vi "Generate Intensities.vi"(9 "eta*cosalpha":dbl=-0.0303, 10 "Lorentzian Width":dbl=0.05, 11 "Numeric":dbl) -> (3 "Intensity":dbl)   [LabVIEW 2020]
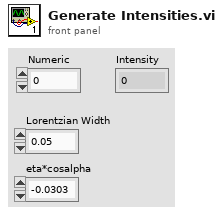
[diagram p1: front panel]
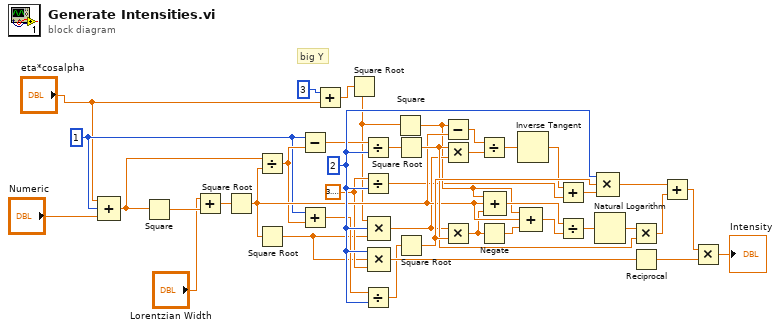
[diagram p0: block diagram]
diagram:
  w18 = 3.141592653589793
  w35 = 2
  w15 = 1
  # "big Y"
  n1 = Compound Arithmetic op=ADD("eta*cosalpha", w15, "Numeric") -> (w9:dbl)
  n2 = Square(x=w9) -> (x^2=w7:dbl)
  n3 = Add(x="Lorentzian Width", y=w7) -> (x+y=w8:dbl)
  n4 = Square Root(x=w8) -> (sqrt(x)=w29:dbl)
  n5 = Divide(x=w9, y=w29) -> (x/y=w16:dbl)
  n6 = Square Root(x=w29) -> (sqrt(x)=w3:dbl)
  n7 = Subtract(x=w15, y=w16) -> (x-y=w11:dbl)
  n8 = Add(x=w15, y=w16) -> (x+y=w10:dbl)
  n9 = Add(x=3, y="eta*cosalpha") -> (x+y=w19:dbl)
  n10 = Square Root(x=w19) -> (sqrt(x)=w5:dbl)
  n11 = Divide(x=w11, y=w35) -> (x/y=w14:dbl)
  n12 = Divide(x=w18, y=w35) -> (x/y=w24:dbl)
  n13 = Divide(x=w10, y=w35) -> (x/y=w13:dbl)
  n14 = Compound Arithmetic op=MULTIPLY(w5, w35, w3) -> (w27:dbl)
  n15 = Compound Arithmetic op=MULTIPLY(w35, w3, w18) -> (w17:dbl)
  n16 = Square(x=w5) -> (x^2=w26:dbl)
  n17 = Square Root(x=w14) -> (sqrt(x)=w34:dbl)
  n18 = Square Root(x=w13) -> (sqrt(x)=w36:dbl)
  n19 = Subtract(x=w26, y=w29) -> (x-y=w20:dbl)
  n20 = Multiply(x=w34, y=w27) -> (x*y=w21:dbl)
  n21 = Multiply(x=w27, y=w36) -> (x*y=w28:dbl)
  n22 = Divide(x=w20, y=w21) -> (x/y=w22:dbl)
  n23 = Negate(x=w28) -> (-x=w25:dbl)
  n24 = Compound Arithmetic op=ADD(w26, w29, w28) -> (w30:dbl)
  n25 = Inverse Tangent(1:w22) -> (0:w23:dbl)
  n26 = Compound Arithmetic op=ADD(w26, w29, w25) -> (w31:dbl)
  n27 = Add(x=w23, y=w24) -> (x+y=w37:dbl)
  n28 = Divide(x=w30, y=w31) -> (x/y=w32:dbl)
  n29 = Natural Logarithm(1:w32) -> (0:w33:dbl)
  n30 = Compound Arithmetic op=MULTIPLY(w35, w36, w37) -> (w38:dbl)
  n31 = Multiply(x=w33, y=w34) -> (x*y=w39:dbl)
  n32 = Reciprocal(x=w17) -> (1/x=w41:dbl)
  n33 = Add(x=w38, y=w39) -> (x+y=w40:dbl)
  n34 = Multiply(x=w40, y=w41) -> (x*y=→"Intensity":dbl)
